vi "Replace Database Path.vi"(8 "error in (no error)":errorcluster, 11 "Value":variant) -> (0 "error out":errorcluster, 3 "Property Name":string)   [LabVIEW 2023, in "Vires VTD System Explorer.lvlib"]
uses:
  Vires VTD System Explorer.lvlib
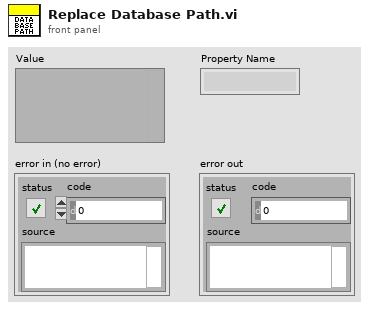
[diagram p1: front panel]
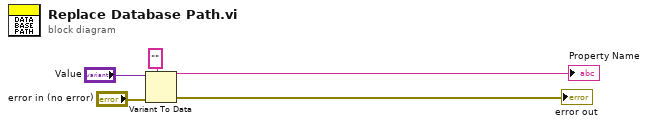
[diagram p0: block diagram]
diagram:
  n1 = Variant To Data(error in="error in (no error)", type="" ("Property Name"), Variant="Value") -> (data=→"Property Name":string, error out=→"error out":errorcluster)
